vi "Write AI Task.vi"(8 "error in (no error)":errorcluster, 10 "AI Task":refnum<k21>, 11 "DAQmx Digitizer in":refnum<class "DAQmx Digitizer.lvclass">) -> (0 "error out":errorcluster, 3 "DAQmx Digitizer out":refnum<class "DAQmx Digitizer.lvclass">)   [LabVIEW 2021, in "DAQmx Digitizer.lvclass"]
uses:
  DAQmx Digitizer.lvclass
  DAQmx Digitizer.lvclass/DAQmx Digitizer.ctl
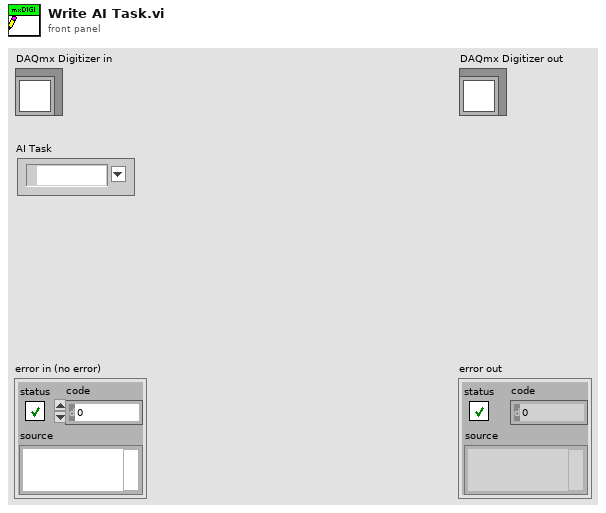
[diagram p1: front panel]
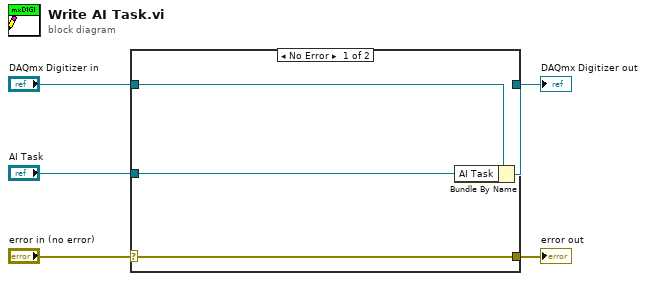
[diagram p0: block diagram]
diagram:
  n1 = case shown="No Error" "error in (no error)" {
    selector: "error in (no error)" -> [w9 w10]
    tunnel: [w9 w10] -> w4
    tunnel: [w7 w11] -> w2
    tunnel: "DAQmx Digitizer in" -> [w8 w11]
    tunnel: "AI Task" -> [w6 _]
    frame No Error {
      n2 = Bundle By Name(cluster=w8, "AI Task"=w6) -> (w7:refnum<class "DAQmx Digitizer.lvclass">)
    }
    frame Error {
    }
  }
  "error out" <- w4
  "DAQmx Digitizer out" <- w2
